vi "Calc_WaveformGenerator.vi"(0 "Scan parameters":T1={"X axis"="1", "Y axis"="2", "# wavepoints"=100, "wave table rate"=10, "area X_min/µm"=0.0, "area Y_min/µm"=2.0, "area Y_max/µm"=8.0, "area X_max/µm"=10.0, "jerk X/pts"=10, "# lines"=4, "bidirectional scan"=TRUE} {"area X_max/µm" format="%.4g"; "area Y_max/µm" format="%.4g"; "area Y_min/µm" format="%.4g"; "area X_min/µm" format="%.4g"}, 1 "Wavepoint":i32[](array[numeric])=[1], 2 "Trigger value 2":i32[](array[numeric])=[1], 5 "System no.":i32=1 min=1 max=4 step=1, 11 "error in 2":errorcluster) -> (4 "wave table rate/ms":dbl=200.0 format="%.3g", 6 "scan time for 1 line/ms":dbl=200.0 format="%.3g", 15 "error out 2":errorcluster)   [LabVIEW 2011]
uses:
  Utilities/controls/ctlSeqFNs_PI_SysNr.ctl
panel:
  in  "No.of digits":i16=1
  in  "Connected Axis":string[](array[string])
  in  "wavepoints":i32
  in  "N":i32
  in  "SegmentLengt":i32
  in  "X0":i32
  in  "SpeedUpDown":dbl
  out "Parameter value 5":dbl[](array[numeric]) format="%.6f"
  out "Hidden error 11":bool
  out "Parameter value 4":dbl[](array[numeric]) format="%.6f"
  out "Hidden error 10":bool
  out "Parameter value 2":dbl[](array[numeric]) format="%.6f"
  out "Hidden error 8":bool
  in  "Trigger value":i32[](array[numeric])
  out "WAV Parameter value":dbl[](array[numeric]) format="%.6f"
  in  "DeviceNr.":T2=enum."E710"
  out "WG running?":bool[](array[boolean])
  out "WGO parameter":i32[](array[numeric])
  in  "TriggerLineCam":dbl[](array[numeric])
  out "spa out":dbl[](array[numeric]) format="%.6f"
  in  "divident":dbl
  out "Command level":i32
  in  "pixel length":dbl
  in  "pixel-start":dbl
  out "Hidden error 6":bool
  out "Hidden error 5":bool
  out "Hidden error 4":bool
  out "Hidden error 3":bool
  in  "error in":errorcluster
  out "Hidden error 2":bool
  out "Hidden error":bool
  out "Wave storage max.":dbl[](array[numeric])
  out "error out":errorcluster
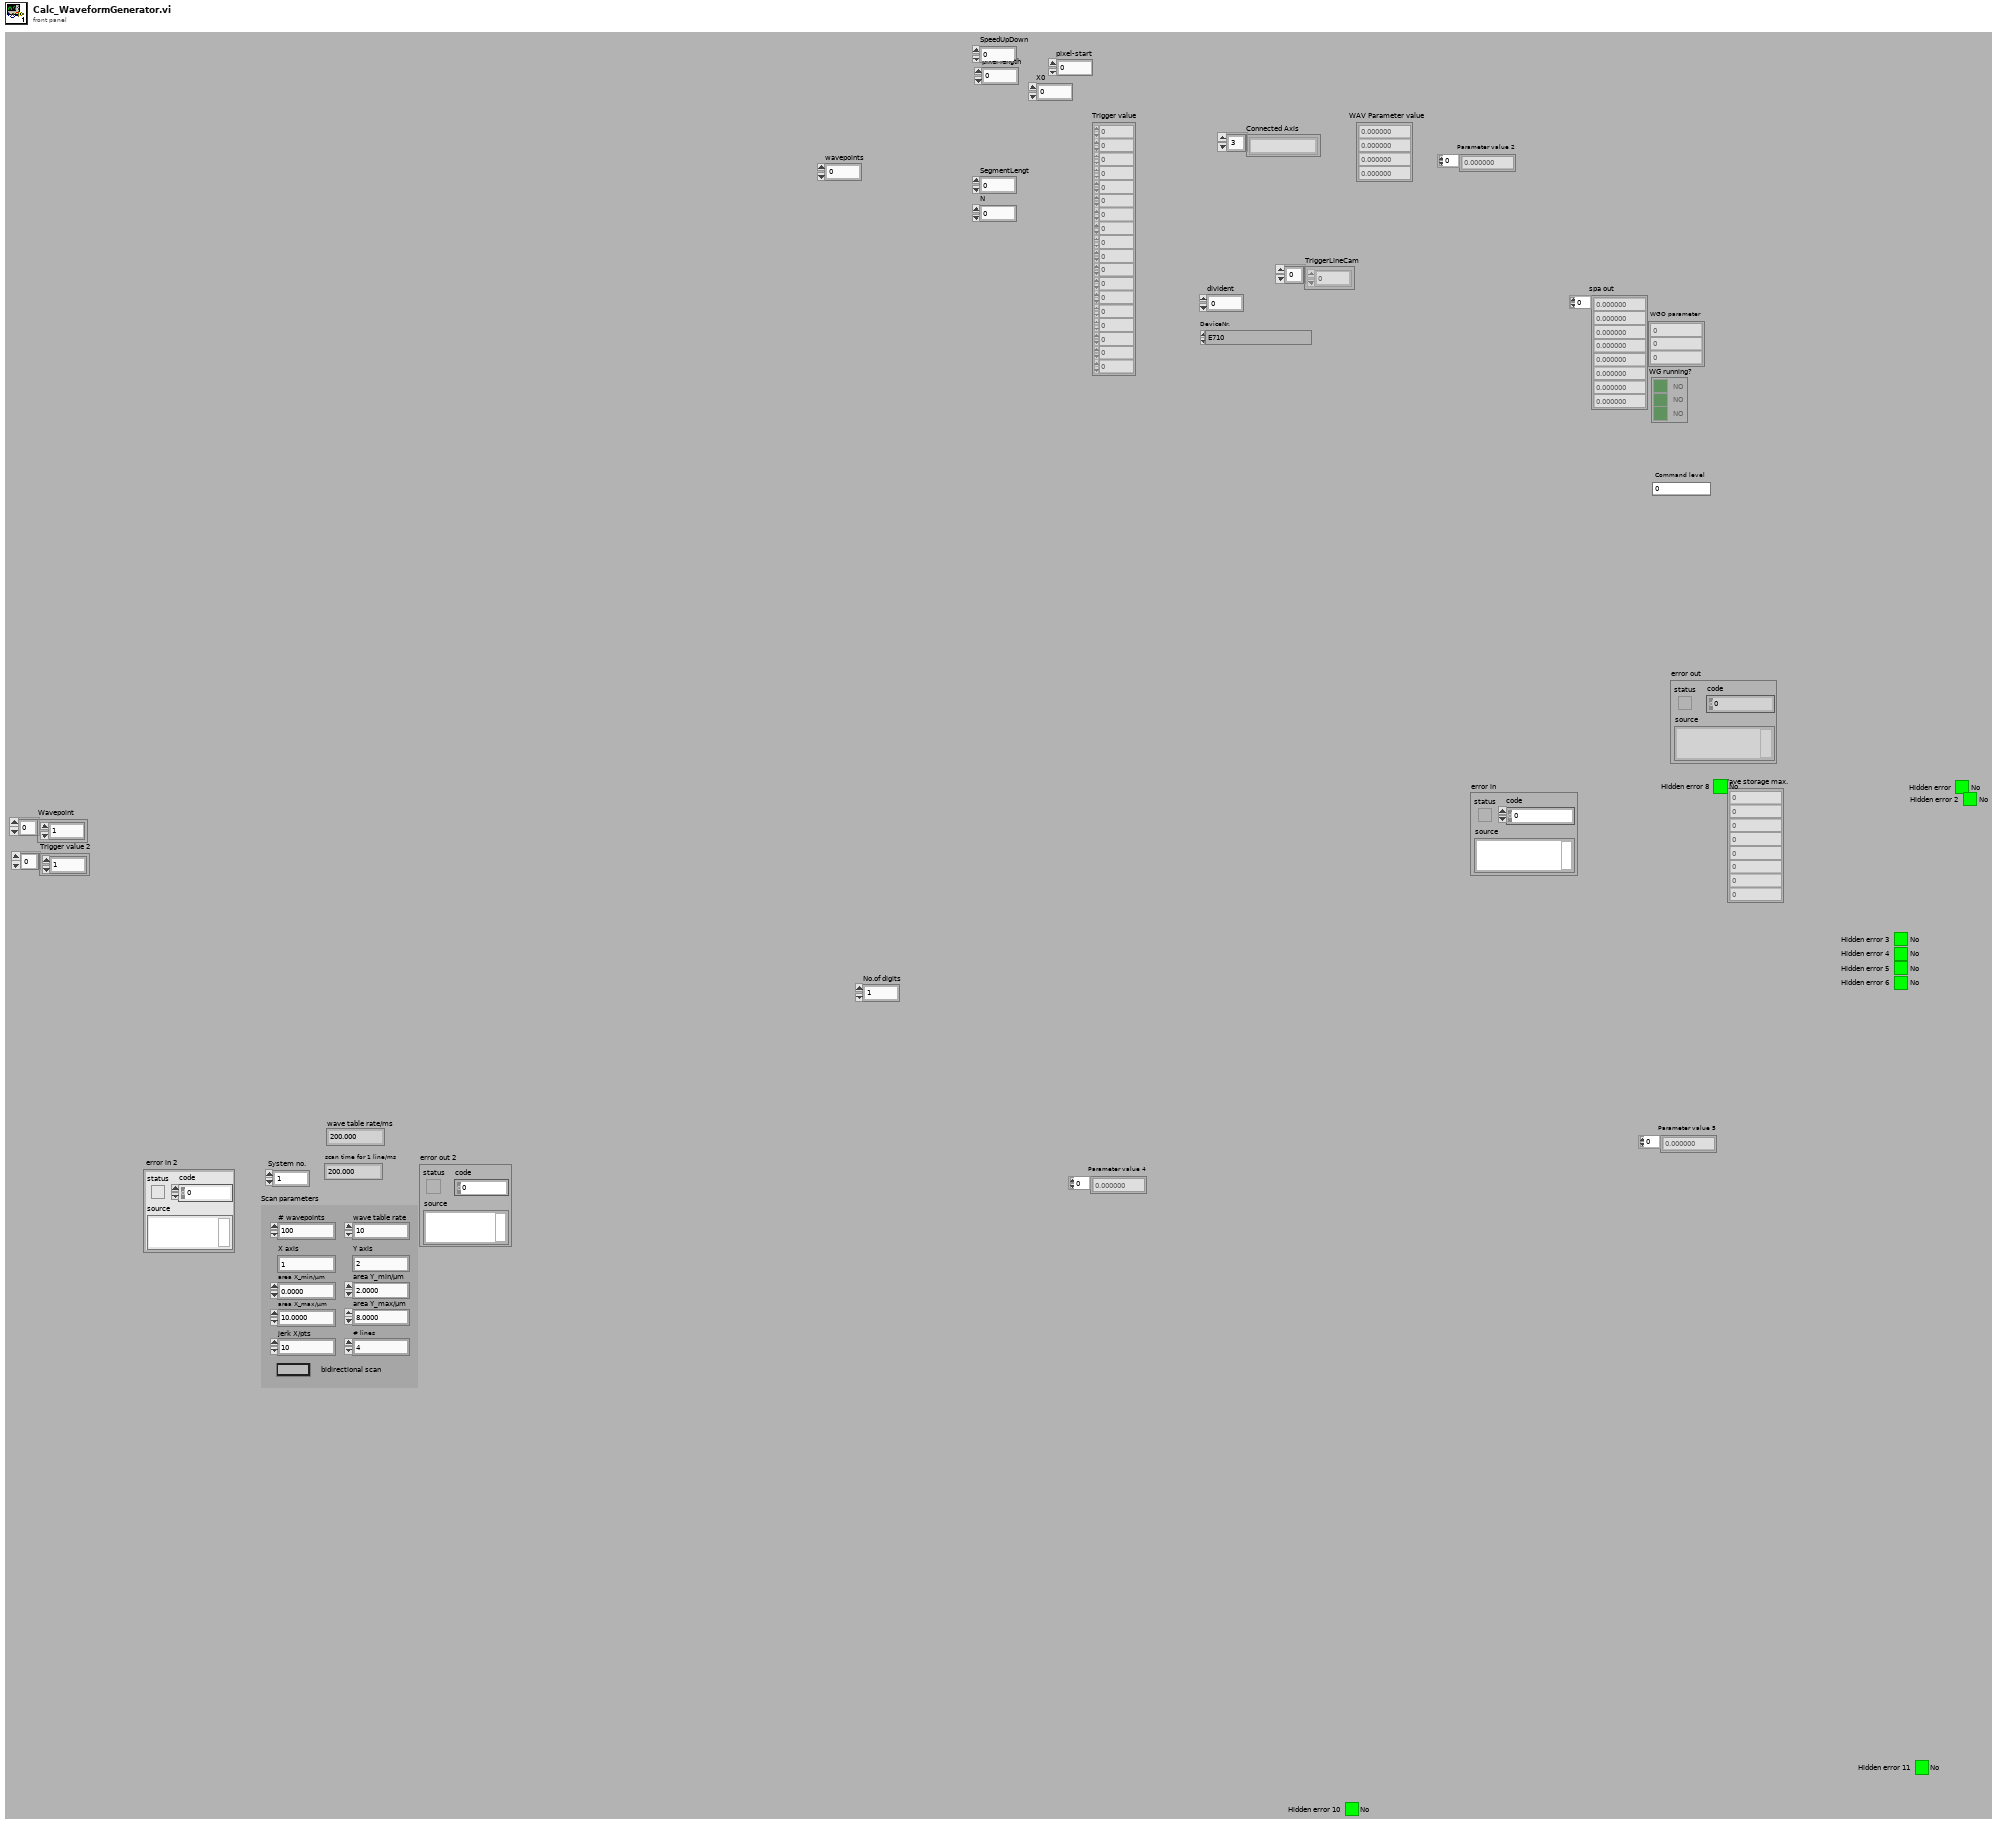
[diagram p1: front panel]
types:
  T1 = cluster{"X axis":string, "Y axis":string, "# wavepoints":i32, "wave table rate":i32, "area X_min/µm":dbl, "area Y_min/µm":dbl, "area Y_max/µm":dbl, "area X_max/µm":dbl, "jerk X/pts":i32, "# lines":i32, "bidirectional scan":bool}
  T2 = typedef "ctlSeqFNs_PI_SysNr.ctl" = enum16{"Zero", "E517", "E710"}
  T3 = cluster{"SpeedUpDown":dbl, "pixel length":dbl, "pixel-start":dbl}
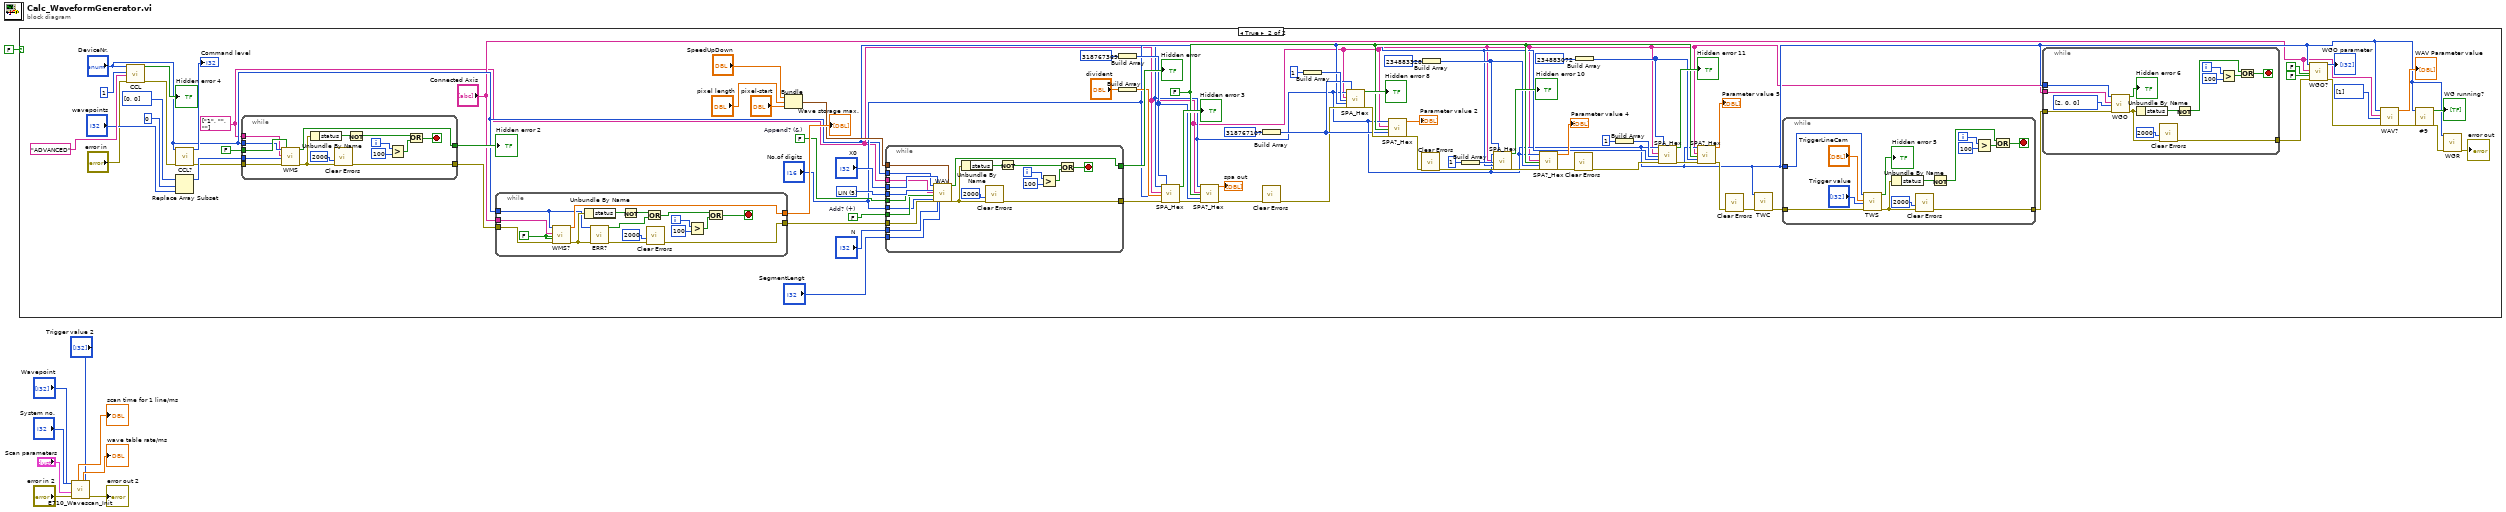
[diagram p0: block diagram]
diagram:
  n1 = case shown="True" FALSE ("Boolean") {
    frame False {
    }
    frame True {
      w15 = string[] ["1", "", ""] ("Affected axes")
      w31 = FALSE ("Without designators?")
      w77 = FALSE  # Add? (+)
      w88 = FALSE  # Append? (&)
      w89 = u16 5 items=["SIN", "POL", "TAN", "PNT", "SIN_P", "LIN", "RAMP"] ("Waveform")
      n2 = call "CCL.vi"("System no."="DeviceNr.", "Command level"=1, "Password"="ADVANCED", "error in"="error in") -> ("Controller error"=→"Hidden error 4":bool, "error out"=w75:errorcluster)  [unwired: 14 in]
      n3 = call "CCL?.vi"("System no."="DeviceNr.", "error in"=w75) -> ("Command level"=→"Command level":i32, "error out"=w12:errorcluster)  [unwired: 16 in]
      n4 = Replace Array Subset(array=i32[] [0, 0] ("Wave storage max. 2"), new element="wavepoints", index=0) -> (w23:i32[])
      n5 = while {
        tunnel: FALSE ("Without axis ID?") -> [w172]
        tunnel: [w171] -> w86
        tunnel: w12 -> [w170]
        tunnel: "DeviceNr." -> [w169]
        tunnel: [w168] -> w18
        tunnel: w23 -> [w159]
        tunnel: w15 -> [w158]
        i -> [w161]
        stop <- w164 stop-if-true
        n6 = call "WMS.vi"("System no."=w169, "Axes to set"=w158, "Wave storage max."=w159, "error in"=w170, "Without axis ID?"=w172) -> ("Controller error"=w171:bool, "error out"=w167:errorcluster)  [unwired: 13 in]
        n7 = Unbundle By Name(w167) -> ("status"=w166:bool)
        n8 = call <vilib>:"Clear Errors.vi"("error in (no error)"=w167, 5:u32 2000 ("milliseconds to wait")) -> ("error out"=w168:errorcluster)  [unwired: 5 in]
        n9 = Not(x=w166) -> (.not. x?=w165:bool)
        n10 = Greater?(x=w161, y=100 ("x")) -> (0:w163:bool)
        n11 = Or(x=w165, y=w163) -> (x .or. y?=w164:bool)
      }
      "Hidden error 2" <- w86
      n12 = while {
        tunnel: [w108] -> w90
        tunnel: "Connected Axis" -> [w107]
        tunnel: "DeviceNr." -> [w92]
        tunnel: w18 -> [w105]
        tunnel: [w94] -> w17
        i -> [w99]
        stop <- w102 stop-if-true
        w106 = FALSE ("All axes?")
        n13 = call "WMS?.vi"("System no."=w92, "Axes to query"=w107, "All axes?"=w106, "Axis identifier?"=w106, "error in"=w105) -> ("Wave storage max."=w108:dbl[], "error out"=w100:errorcluster)  [unwired: 13 in]
        n14 = Unbundle By Name(w100) -> ("status"=w101:bool)
        n15 = call "ERR?.vi"("System no."=w92, "error in"=w100) -> ("Controller error"=w97:bool, "error out"=w95:errorcluster)  [unwired: 16 in]
        n16 = Not(x=w101) -> (.not. x?=w98:bool)
        n17 = Or(x=w98, y=w97) -> (x .or. y?=w96:bool)
        n18 = call <vilib>:"Clear Errors.vi"("error in (no error)"=w95, 5:u32 2000 ("milliseconds to wait")) -> ("error out"=w94:errorcluster)  [unwired: 5 in]
        n19 = Greater?(x=w99, y=100 ("x")) -> (0:w104:bool)
        n20 = Or(x=w96, y=w104) -> (x .or. y?=w102:bool)
      }
      "Wave storage max." <- w90
      n21 = Bundle("SpeedUpDown"="SpeedUpDown", "pixel length"="pixel length", "pixel-start"="pixel-start") -> (w85:T3)  [unwired: 1 in]
      n22 = while {
        tunnel: w17 -> [w129]
        tunnel: w89 -> [w128]
        tunnel: w88 -> [w127]
        tunnel: w77 -> [w126]
        tunnel: [w111] -> w14
        tunnel: [w125] -> w87
        tunnel: w85 -> [w124]
        tunnel: "X0" -> [w123]
        tunnel: "N" -> [w122]
        tunnel: "No.of digits" -> [w121]
        tunnel: "SegmentLengt" -> [w120]
        tunnel: "DeviceNr." -> [w119]
        tunnel: w15 -> [w109]
        i -> [w114]
        stop <- w115 stop-if-true
        n23 = call "WAV.vi"("System no."=w119, "Waveform"=w128, "Affected axes"=w109, "Append? (&)"=w127, "Add? (+)"=w126, "No.of digits"=w121, "error in"=w129, "Xo"=w123, "N"=w122, "Segment length"=w120, "LIN Parameters"=w124) -> ("Controller error"=w125:bool, "error out"=w112:errorcluster)  [unwired: 15 in]
        n24 = Unbundle By Name(w112) -> ("status"=w117:bool)
        n25 = call <vilib>:"Clear Errors.vi"("error in (no error)"=w112, 5:u32 2000 ("milliseconds to wait")) -> ("error out"=w111:errorcluster)  [unwired: 5 in]
        n26 = Not(x=w117) -> (.not. x?=w116:bool)
        n27 = Greater?(x=w114, y=100 ("x")) -> (0:w118:bool)
        n28 = Or(x=w116, y=w118) -> (x .or. y?=w115:bool)
      }
      "Hidden error" <- w87
      n29 = Build Array(u32 318767369 ("new element/subarray")) -> (w60:u32[])
      n30 = Build Array("divident") -> (w64:dbl[])
      n31 = call "SPA_Hex.vi"("System no."="DeviceNr.", "Designator to set"=w15, "Parameter value"=w64, "No.of digits"="No.of digits", "error in"=w14, "Parameter number (hex)"=w60) -> ("Controller error"=→"Hidden error 3":bool, "error out"=w63:errorcluster)  [unwired: 12 in]
      n32 = call "SPA?_Hex.vi"("System no."="DeviceNr.", "Designator to query"=w15, "Without designators?"=w31, "Parameter no. (hex)"=w60, "error in"=w63) -> ("Parameter value"=→"spa out":dbl[], "error out"=w59:errorcluster)  [unwired: 13 in]
      n33 = Build Array(u32 318767107 ("new element/subarray")) -> (w51:u32[])
      n34 = call <vilib>:"Clear Errors.vi"("error in (no error)"=w59) -> ("error out"=w32:errorcluster)  [unwired: 6 in]
      n35 = Build Array(1 ("new element/subarray")) -> (w52:i32[])
      n36 = call "SPA_Hex.vi"("System no."="DeviceNr.", "Designator to set"=w15, "Parameter value"=w52, "No.of digits"="No.of digits", "error in"=w32, "Parameter number (hex)"=w51) -> ("Controller error"=→"Hidden error 8":bool, "error out"=w58:errorcluster)  [unwired: 12 in]
      n37 = call "SPA?_Hex.vi"("System no."="DeviceNr.", "Designator to query"=w15, "Without designators?"=w31, "Parameter no. (hex)"=w51, "error in"=w58) -> ("Parameter value"=→"Parameter value 2":dbl[], "error out"=w56:errorcluster)  [unwired: 13 in]
      n38 = call <vilib>:"Clear Errors.vi"("error in (no error)"=w56) -> ("error out"=w33:errorcluster)  [unwired: 6 in]
      n39 = Build Array(u32 234883328 ("new element/subarray")) -> (w43:u32[])
      n40 = Build Array(1 ("new element/subarray")) -> (w44:i32[])
      n41 = call "SPA_Hex.vi"("System no."="DeviceNr.", "Designator to set"=w15, "Parameter value"=w44, "No.of digits"="No.of digits", "error in"=w33, "Parameter number (hex)"=w43) -> ("Controller error"=→"Hidden error 10":bool, "error out"=w50:errorcluster)  [unwired: 12 in]
      n42 = call "SPA?_Hex.vi"("System no."="DeviceNr.", "Designator to query"=w15, "Without designators?"=w31, "Parameter no. (hex)"=w43, "error in"=w50) -> ("Parameter value"=→"Parameter value 4":dbl[], "error out"=w48:errorcluster)  [unwired: 13 in]
      n43 = call <vilib>:"Clear Errors.vi"("error in (no error)"=w48) -> ("error out"=w34:errorcluster)  [unwired: 6 in]
      n44 = Build Array(u32 234883072 ("new element/subarray")) -> (w35:u32[])
      n45 = Build Array(i16 1 ("new element/subarray")) -> (w36:i16[])
      n46 = call "SPA_Hex.vi"("System no."="DeviceNr.", "Designator to set"=w15, "Parameter value"=w36, "No.of digits"="No.of digits", "error in"=w34, "Parameter number (hex)"=w35) -> ("Controller error"=→"Hidden error 11":bool, "error out"=w42:errorcluster)  [unwired: 12 in]
      n47 = call "SPA?_Hex.vi"("System no."="DeviceNr.", "Designator to query"=w15, "Without designators?"=w31, "Parameter no. (hex)"=w35, "error in"=w42) -> ("Parameter value"=→"Parameter value 5":dbl[], "error out"=w40:errorcluster)  [unwired: 13 in]
      n48 = call <vilib>:"Clear Errors.vi"("error in (no error)"=w40) -> ("error out"=w11:errorcluster)  [unwired: 6 in]
      n49 = call "TWC.vi"("System no."="DeviceNr.", "error in"=w11) -> ("error out"=w10:errorcluster)  [unwired: 17 in]
      n50 = while {
        tunnel: [w152] -> w76
        tunnel: "DeviceNr." -> [w155]
        tunnel: w10 -> [w144]
        i -> [w154]
        stop <- w146 stop-if-true
        n51 = call "TWS.vi"("System no."=w155, "Wavepoint"="TriggerLineCam", "Trigger value"="Trigger value", "error in"=w144) -> ("Controller error"=→"Hidden error 5":bool, "error out"=w148:errorcluster)  [unwired: 14 in]
        n52 = Unbundle By Name(w148) -> ("status"=w150:bool)
        n53 = call <vilib>:"Clear Errors.vi"("error in (no error)"=w148, 5:u32 2000 ("milliseconds to wait")) -> ("error out"=w152:errorcluster)  [unwired: 5 in]
        n54 = Not(x=w150) -> (.not. x?=w149:bool)
        n55 = Greater?(x=w154, y=100) -> (0:w147:bool)
        n56 = Or(x=w149, y=w147) -> (x .or. y?=w146:bool)
      }
      n57 = while {
        tunnel: [w133] -> w83
        tunnel: w76 -> [w135]
        tunnel: "DeviceNr." -> [w141]
        tunnel: w15 -> [w130]
        i -> [w132]
        stop <- w136 stop-if-true
        n58 = call "WGO.vi"("System no."=w141, "Affected axes"=w130, "WGO Parameter"=i32[] [2, 0, 0], "error in"=w135) -> ("Controller error"=→"Hidden error 6":bool, "error out"=w131:errorcluster)  [unwired: 14 in]
        n59 = Unbundle By Name(w131) -> ("status"=w139:bool)
        n60 = call <vilib>:"Clear Errors.vi"("error in (no error)"=w131, 5:u32 2000 ("milliseconds to wait")) -> ("error out"=w133:errorcluster)  [unwired: 5 in]
        n61 = Not(x=w139) -> (.not. x?=w138:bool)
        n62 = Greater?(x=w132, y=100) -> (0:w137:bool)
        n63 = Or(x=w138, y=w137) -> (x .or. y?=w136:bool)
      }
      n64 = call "WGO?.vi"("System no."="DeviceNr.", "Axes to query"="Connected Axis", "All axes?"=FALSE, "Axis identifier?"=FALSE, "error in"=w83) -> ("WGO parameter"=→"WGO parameter":i32[], "error out"=w69:errorcluster)  [unwired: 13 in]
      n65 = call "WAV?.vi"("System no."="DeviceNr.", "Axes to query"="Connected Axis", "Parameter no."=i32[] [1], "error in"=w69) -> ("WAV Parameter value"=→"WAV Parameter value":dbl[], "error out"=w68:errorcluster)  [unwired: 14 in]
      n66 = call "#9.vi"("System no."="DeviceNr.", "error in"=w68) -> ("WG running?"=→"WG running?":bool[], "error out"=w78:errorcluster)  [unwired: 16 in]
      n67 = call "WGR.vi"("System no."="DeviceNr.", "error in"=w78) -> ("error out"=→"error out":errorcluster)  [unwired: 17 in]
    }
  }
  n68 = call <userlib>:"E710_Wavescan_Init.vi"(2:"Trigger value 2", 3:"Wavepoint", "error in"="error in 2", "Scan parameters"="Scan parameters", "System no."="System no.") -> ("error out"=→"error out 2":errorcluster, "wave table rate/ms"=→"wave table rate/ms":dbl, "scan time for 1 line/ms"=→"scan time for 1 line/ms":dbl)  [unwired: 4 in]
